vi "Live window-Event handler-slider menu activ.vi"(7 "Left/Right":T1, 11 "Image intensity slider Menu":refnum<k9>) -> ()   [LabVIEW 2013]
uses:
  Typedefs/Left-Right enum.ctl
  Globals/gl_Windows Ctrl refs.vi
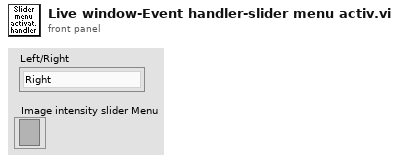
[diagram p1: front panel]
types:
  T1 = typedef "Left-Right enum.ctl" = enum16{"Right", "Left"}
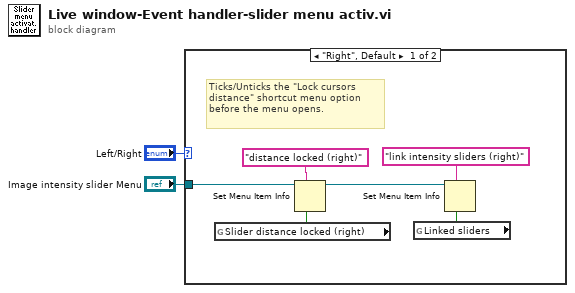
[diagram p0: block diagram]
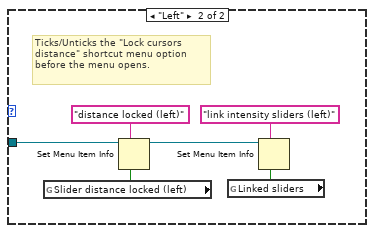
[diagram p2: hidden frame]
diagram:
  n1 = case shown="\"Right\", Default" "Left/Right" {
    tunnel: "Image intensity slider Menu" -> [w6 w14]
    frame "Right", Default {
      # "Ticks/Unticks the \"Lock cursors distance\" shortcut menu option before the menu opens."
      n2 = global read "gl_Windows Ctrl refs.vi" "Slider distance locked (right)"() -> (w7:bool)
      n3 = Set Menu Item Info(6:w7, 7:"distance locked (right)", 11:w6) -> (3:w3:refnum<k9>)  [unwired: 4 in, 1 out]
      n4 = global read "gl_Windows Ctrl refs.vi" "Linked sliders"() -> (w5:bool)
      n5 = Set Menu Item Info(6:w5, 7:"link intensity sliders (right)", 11:w3) -> ()  [unwired: 4 in, 2 out]
    }
    frame "Left" {
      # "Ticks/Unticks the \"Lock cursors distance\" shortcut menu option before the menu opens."
      n6 = global read "gl_Windows Ctrl refs.vi" "Slider distance locked (left)"() -> (w13:bool)
      n7 = Set Menu Item Info(6:w13, 7:"distance locked (left)", 11:w14) -> (3:w11:refnum<k9>)  [unwired: 4 in, 1 out]
      n8 = global read "gl_Windows Ctrl refs.vi" "Linked sliders"() -> (w10:bool)
      n9 = Set Menu Item Info(6:w10, 7:"link intensity sliders (left)", 11:w11) -> ()  [unwired: 4 in, 2 out]
    }
  }
